vi "xiC - DeferPanelUpdate.vi"(6 "Operand":enum16{"Lock", "Release"}(ring), 8 "error in (no error)":errorcluster, 11 "Attributes":T1) -> (0 "error out":errorcluster, 3 "Attributes":T1)   [LabVIEW 2013]
uses:
  xiC - Attributes.ctl
  C:/Projects/Cameras3.x/xiLib/xiLIB_64bit/xiLIB/xiCamLib/API/x64/xiApi.NETX64.dll
  xiLIB_64bit/xiLIB/xiCamLib/API/x64/xiApi.NETX64.dll
  xiC - TreeDisplayType.ctl
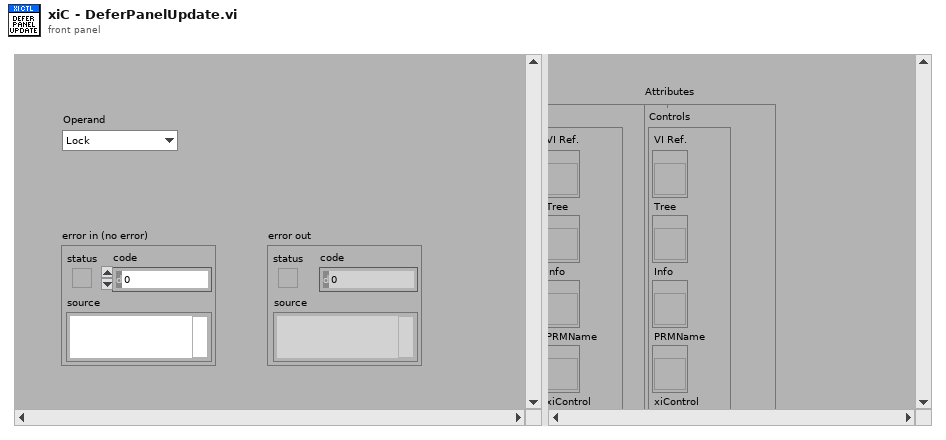
[diagram p1: front panel]
types:
  T1 = typedef "xiC - Attributes.ctl" = cluster{"Controls":cluster{"VI Ref.":refnum<vi>, "Tree":refnum<vi>, "Info":refnum<vi>, "PRMName":refnum<vi>, "xiControl":refnum<vi>, "Error":refnum<vi>, "SW_TRG":refnum<vi>, "ImageDisplay":refnum<vi>}, "Variables":cluster{"ProcessQ.":refnum<queue>, "Data":bool, "xiCam":refnum<k24>, "Tree_Display_Type":T2}}
  T2 = typedef "xiC - TreeDisplayType.ctl" = enum16{"DEFAULT", "HIDE_MAX_MIN"}
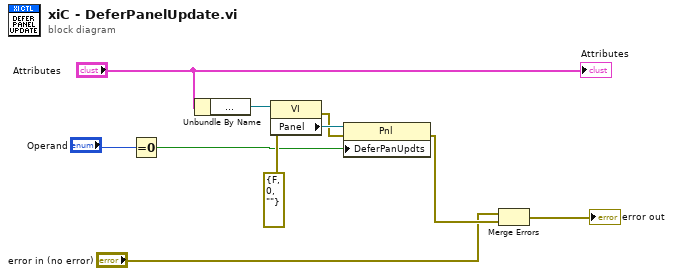
[diagram p0: block diagram]
diagram:
  n1 = Equal To 0?(x="Operand") -> (x = 0?=w4:bool)
  n2 = Unbundle By Name("Attributes") -> ("Controls.VI Ref."=w9:refnum<vi>)
  n3 = property class="VI"(reference=w9, error in=errorcluster {"status"=FALSE, "code"=0, "source"=""} ("error in (no error)")) -> (error out=w6:errorcluster, "Panel"=w8:refnum<vi>)  [unwired: 1 out]
  n4 = property class="Pnl"(reference=w8, error in=w6, "DeferPanUpdts"=w4) -> (error out=w3:errorcluster)  [unwired: 1 out]
  n5 = Merge Errors("error in (no error)", w3) -> (→"error out":errorcluster)
  "Attributes" <- "Attributes"
